vi "dummyfpga.vi"() -> ()   [LabVIEW 2017]
panel:
  in  "Numeric":i16
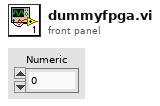
[diagram p1: front panel]
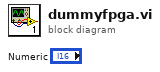
[diagram p0: block diagram]
diagram:
